vi "LLP Packet Acquisition Loop.vi"(0 "fpga interface in":refnum<k20>, 1 "bytes acquired references":refnum<vi>[](array[refnum]), 5 "Serial Channels":string[](array[string]), 7 "tdms file directory":path, 9 "display acquired packets":bool=TRUE, 11 "error in":errorcluster, 12 "log to disk":bool=TRUE, 13 "num packets to read":i64=-1) -> (4 "number of packets acquired":i64[](array[numeric]), 6 "number of bytes acquired":i64[](array[numeric]), 8 "display data":string[][][](array[string]), 15 "error out":errorcluster)   [LabVIEW 2025, in "GettingStarted_Acq_148X_Host.lvlib"]
uses:
  GettingStarted_Acq_148X_Host.lvlib
  Common/GettingStarted_Common_148X_Host.lvlib
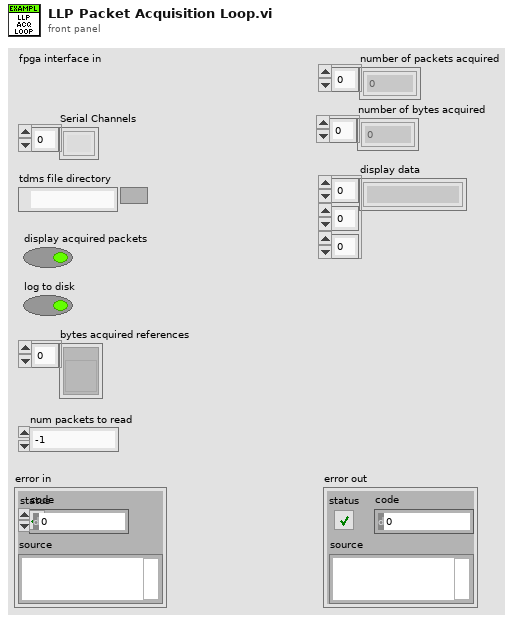
[diagram p1: front panel]
types:
  T1 = typedef "NI CSI-2 API Host v2.lvlib/Host Tagged LLP Packet.ctl" = cluster{"tag":T2, "llp packet":T6}
  T2 = typedef "NI CSI-2 API Host v2.lvlib/Host LLP Packet Tag.ctl" = cluster{"timestamp":T3, "size":T5}
  T3 = typedef "NI CSI-2 API Host v2.lvlib/Host LLP Packet Timestamp.ctl" = cluster{"valid":bool, "count":u64, "id":T4, "metadata":u8}
  T4 = typedef "NI CSI-2 API FPGA v2.lvlib/Timestamp ID.ctl" = enum8{"SI0 LLP", "SI1 LLP", "SI2 LLP", "SI3 LLP", "SI4 LLP", "SI5 LLP", "SI6 LLP", "SI7 LLP", "SO0 LLP", "SO1 LLP", "SO2 LLP", "SO3 LLP", "SO4 LLP", "SO5 LLP", "SO6 LLP", "SO7 LLP", "Ser0 GPIO Bank", "Ser1 GPIO Bank", "Ser2 GPIO Bank", "Ser3 GPIO Bank", "Ser4 GPIO Bank", "Ser5 GPIO Bank", "Ser6 GPIO Bank", "Ser7 GPIO Bank", "Des0 GPIO Bank", "Des1 GPIO Bank", "Des2 GPIO Bank", "Des3 GPIO Bank", "Des4 GPIO Bank", "Des5 GPIO Bank", "Des6 GPIO Bank", "Des7 GPIO Bank", "User0", "User1", "User2", "User3", "User4", "User5", "User6", "User7", "User8", "User9", "User10", "User11", "User12", "User13", "User14", "User15", "User16", "User17", "User18", "User19", "User20", "User21", "User22", "User23", "User24", "User25", "User26", "User27", "User28", "User29", "User30", "User31"}
  T5 = typedef "NI CSI-2 API Host v2.lvlib/Host LLP Packet Size.ctl" = cluster{"bytes":u32, "valid":bool}
  T6 = typedef "NI CSI-2 API Host v2.lvlib/Host LLP Packet.ctl" = cluster{"header":T7, "payload":u8[], "footer":T8}
  T7 = typedef "NI CSI-2 API FPGA v2.lvlib/LLP Packet Header.ctl" = cluster{"word count":u16, "ecc":fxp<+,6,6>, "vcx":fxp<+,2,2>, "data type":fxp<+,6,6>, "vc":fxp<+,2,2>}
  T8 = typedef "NI CSI-2 API FPGA v2.lvlib/LLP Packet Footer.ctl" = cluster{"crc":u16}
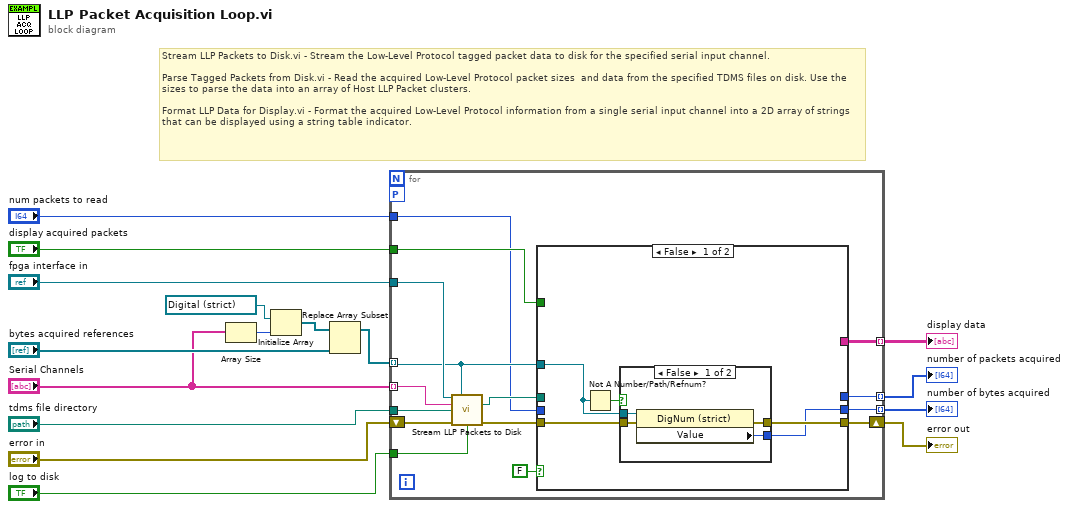
[diagram p0: block diagram]
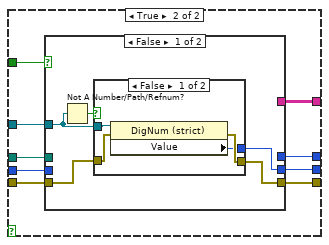
[diagram p3: hidden frame]
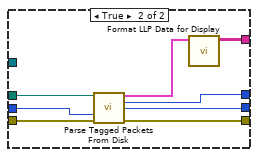
[diagram p5: hidden frame]
diagram:
  # "Stream LLP Packets to Disk.vi - Stream the Low-Level Protocol tagged packet data to disk for the specified serial input channel.\n\nParse Tagged Packets from Disk.vi - Read the acquired Low-Level Protocol packet sizes  and data from the specified TDMS files on disk. Use the sizes to parse the data into an array of Host LLP Packet clusters.\n\nFormat LLP Data for Display.vi - Format the acquired Low-Level Protocol information from a single serial input channel into a 2D array of strings that can be displayed using a string table indicator."
  n1 = Array Size(array="Serial Channels") -> (size(s)=w12:i32)
  n2 = Initialize Array(refnum<vi> refnum ("Number of Bytes Acquired"), w12) -> (w13:refnum<vi>[])
  n3 = Replace Array Subset(array=w13, new element="bytes acquired references") -> (w15:refnum<vi>[])  [unwired: 1 in]
  n4 = for {
    tunnel: [w31] -> w8 mode=indexing
    tunnel: [w23] -> w9 mode=indexing
    tunnel: "Serial Channels" -> [w28] mode=indexing
    tunnel: "fpga interface in" -> [w27]
    shift-right: [w20] -> w7
    shift-left: "error in" -> [w26]
    tunnel: "display acquired packets" -> [w30]
    workers-P: _ -> [_]
    tunnel: "tdms file directory" -> [w29]
    tunnel: w15 -> [w19] mode=indexing
    tunnel: "log to disk" -> [w25]
    tunnel: [w21] -> w3 mode=indexing
    tunnel: "num packets to read" -> [w18]
    n5 = call "Stream LLP Packets to Disk.vi"("fpga interface in"=w27, "bytes acquired indicator ref"=w19, "serial input channel"=w28, "base packet file path"=w29, "error in (no error)"=w26, "log to disk"=w25) -> ("file path out"=w24:path, "error out"=w22:errorcluster)  [unwired: 6 in, 2 out]
    n6 = case shown="False" FALSE {
      tunnel: [_ w50] -> w31
      tunnel: [_ w45] -> w23
      tunnel: [w34 w49] -> w20
      tunnel: w24 -> [_ w48]
      tunnel: w22 -> [w35 w47]
      tunnel: w30 -> [_ w46]
      tunnel: [w33 w44] -> w21
      tunnel: w19 -> [w32 w43]
      tunnel: w18 -> [_ w42]
      frame False {
        n7 = Not A Number/Path/Refnum?(number/path/refnum=w32) -> (NaN/Path/Refnum?=w36:bool)
        n8 = case shown="False" w36 {
          tunnel: [w40 w41] -> w34
          tunnel: [w39 _] -> w33
          tunnel: w35 -> [w38 w41]
          tunnel: w32 -> [w37 _]
          frame False {
            n9 = property class="DigNum (strict)"(reference=w37, error in=w38) -> (error out=w40:errorcluster, "Value"=w39:i64)  [unwired: 1 out]
          }
          frame True {
          }
        }
      }
      frame True {
        n10 = case shown="False" w46 {
          tunnel: [_ w68] -> w50
          tunnel: [_ w63] -> w45
          tunnel: [w54 w64] -> w49
          tunnel: w48 -> [_ w67]
          tunnel: w47 -> [w55 w65]
          tunnel: [w52 w62] -> w44
          tunnel: w43 -> [w51 _]
          tunnel: w42 -> [_ w61]
          frame False {
            n11 = Not A Number/Path/Refnum?(number/path/refnum=w51) -> (NaN/Path/Refnum?=w53:bool)
            n12 = case shown="False" w53 {
              tunnel: [w59 w60] -> w54
              tunnel: [w58 _] -> w52
              tunnel: w51 -> [w57 _]
              tunnel: w55 -> [w56 w60]
              frame False {
                n13 = property class="DigNum (strict)"(reference=w57, error in=w56) -> (error out=w59:errorcluster, "Value"=w58:i64)  [unwired: 1 out]
              }
              frame True {
              }
            }
          }
          frame True {
            n14 = call "Parse Tagged Packets From Disk.vi"("llp tagged packet file path"=w67, "num packets to read"=w61, "error in"=w65) -> ("tagged packets"=w66:T1[], "total packets in file"=w63:i64, "total tagged packet bytes in file"=w62:i64, "error out"=w64:errorcluster)  [unwired: 9 in]
            n15 = call "Format LLP Data for Display.vi"("tagged packets"=w66) -> ("display data"=w68:string[][])  [unwired: 10 in]
          }
        }
      }
    }
  }
  "number of packets acquired" <- w9
  "display data" <- w8
  "error out" <- w7
  "number of bytes acquired" <- w3
